vi "Query Supported Ranges and Sensor Excitation Values.vi"(10 "AI measurement type":i32, 11 "active device":tag) -> (0 "sensor excitation label":string, 1 "AI ranges":dbl[](array[numeric]), 2 "sensor excitation values":dbl[](array[numeric]), 3 "AI couplings":i32[](array[numeric]))   [LabVIEW 2016]
uses:
  <resource>/objmgr/daqmx.rc
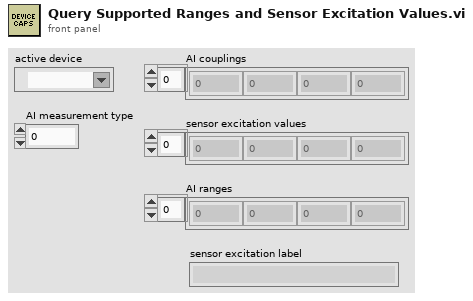
[diagram p1: front panel]
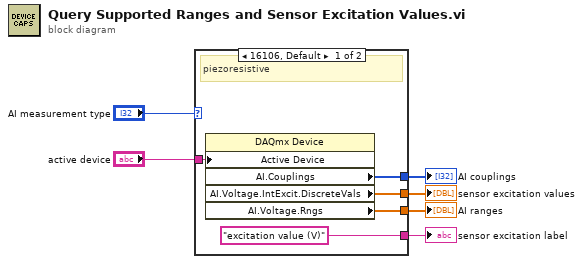
[diagram p0: block diagram]
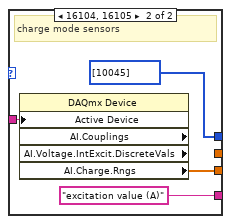
[diagram p2: hidden frame]
diagram:
  n1 = case shown="16106, Default" "AI measurement type" {
    tunnel: [w9 w15] -> w1
    tunnel: [w10 _] -> w2
    tunnel: [w7 w12] -> w3
    tunnel: "active device" -> [w11 w14]
    tunnel: ["excitation value (V)" ("regular expression") "excitation value (A)" ("regular expression")] -> w6
    frame 16106, Default {
      # "piezoresistive"
      n2 = property class="DAQmx Device"("Active Device"=w11) -> ("AI.Couplings"=w7:i32[], "AI.Voltage.IntExcit.DiscreteVals"=w10:dbl[], "AI.Voltage.Rngs"=w9:dbl[])  [unwired: 2 in, 2 out]
    }
    frame 16104, 16105 {
      w12 = i32[] [10045] items=["Default"=0, "AC"=10045, "DC"=10050, "GND"=10066] ("AI.Couplings")
      # "charge mode sensors"
      n3 = property class="DAQmx Device" props=["Active Device", "AI.Couplings", "AI.Voltage.IntExcit.DiscreteVals", "AI.Charge.Rngs"]("Active Device"=w14) -> ("AI.Charge.Rngs"=w15:dbl[])  [unwired: 2 in, 4 out]
    }
  }
  "sensor excitation label" <- w6
  "AI couplings" <- w3
  "sensor excitation values" <- w2
  "AI ranges" <- w1
